vi "Opgave 6.2 2015 udgave.vi"() -> ()   [LabVIEW 2015]
doc: "This VI is a solution to an exercise in the LabVIEW Basics I course.\n\nThis VI concatenates a message string, a number, and a unit string and writes it to a file."
panel:
  out "File Path":path
  in  "Unit to Write":string="Volts"
  in  "Number to Write":dbl=12.45 format="%.2f"
  in  "String to Write":string="The measurement is:"
  # "*path indicator*"
  # "*string control*\nShow the Scrollbar"
  # "*digital control*"
  # "*string control*"
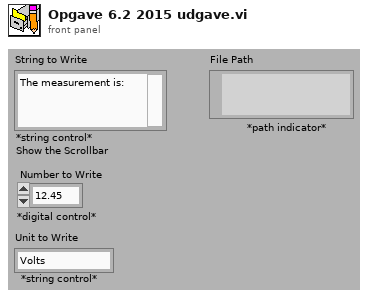
[diagram p1: front panel]
types:
  T1 = enum16{"open", "open or create", "create or replace", "create", "open (read only)"}
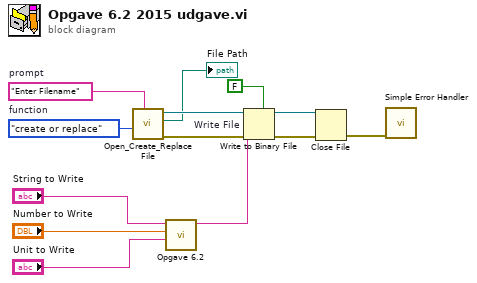
[diagram p0: block diagram]
diagram:
  w12 = T1."create or replace"  # function
  w13 = "Enter Filename"  # prompt
  n1 = call <vilib>:"Open_Create_Replace File.vi"("prompt"=w13, "function (open:0)"=w12) -> ("error out"=w7:errorcluster, "new file path"=→"File Path":path, "refnum"=w11:refnum<file>)  [unwired: 6 in, 1 out]
  n2 = call "Opgave 6.2.vi"("Trailer"="Unit to Write", "Number"="Number to Write", "Header"="String to Write") -> ("Combined String"=w6:string)  [unwired: 1 in, 3 out]
  n3 = Write to Binary File "Write File"(file (use dialog)=w11, data=w6, error in=w7, 5:FALSE ("prepend array or string size? (T)")) -> (refnum out=w10:refnum<file>, error out=w8:errorcluster)  [unwired: 2 in, 1 out]
  n4 = Close File(refnum=w10, error in=w8) -> (error out=w9:errorcluster)  [unwired: 1 out]
  n5 = call <vilib>:"Simple Error Handler.vi"("error in (no error)"=w9) -> ()  [unwired: 4 in, 5 out]
